vi "Práctica01_Ejercicio1_1.vi"() -> ()   [LabVIEW 2020]
panel:
  out "Boolean 5":bool
  in  "Latch Until Released\nAntes de correr el programa presionalo\ndespues correlo una sola vez y observa el resultado cambia solo si esta presionado":bool
  out "Boolean 3":bool
  in  "Latch when Released\nAntes de correr el programa presionalo\ndespues correlo una sola vez y observa el resultado cuando lo sueltas":bool
  out "Boolean":bool
  in  "Latch When Pressed \nAntes de correr el programa presionalo\ndespues correlo una sola vez y observa el resultado enclavado":bool
  out "Boolean 6":bool
  in  "Switch Until Released\nPush button, solo cambia si esta presionado":bool
  out "Boolean 4":bool
  in  "Switch when Released\nCambia cuando lo sueltas":bool
  out "Boolean 2":bool
  in  "Switch when Pressed - \nCambia cuando lo presionas":bool
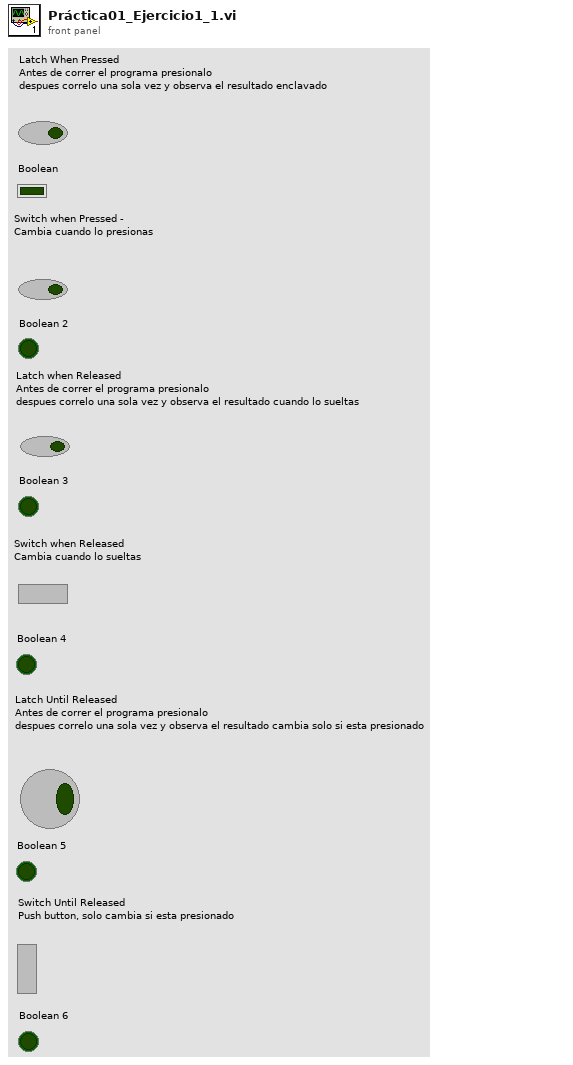
[diagram p1: front panel]
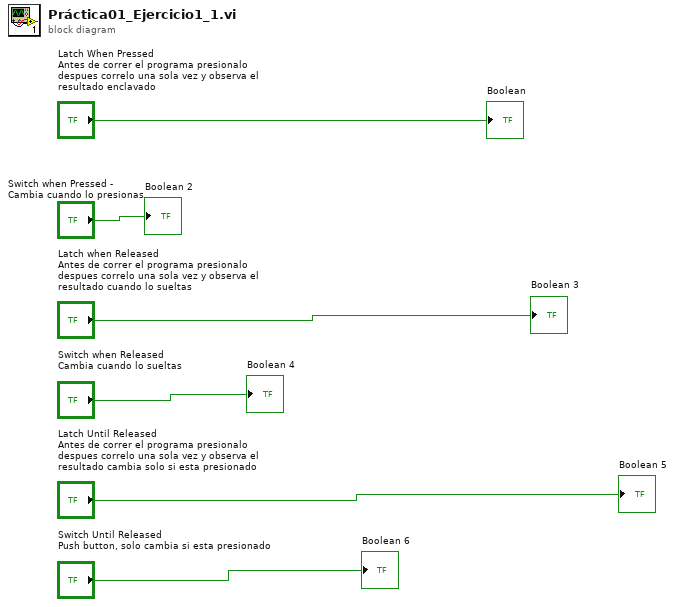
[diagram p0: block diagram]
diagram:
  "Boolean 2" <- "Switch when Pressed - \nCambia cuando lo presionas"
  "Boolean 4" <- "Switch when Released\nCambia cuando lo sueltas"
  "Boolean 6" <- "Switch Until Released\nPush button, solo cambia si esta presionado"
  "Boolean" <- "Latch When Pressed \nAntes de correr el programa presionalo\ndespues correlo una sola vez y observa el resultado enclavado"
  "Boolean 3" <- "Latch when Released\nAntes de correr el programa presionalo\ndespues correlo una sola vez y observa el resultado cuando lo sueltas"
  "Boolean 5" <- "Latch Until Released\nAntes de correr el programa presionalo\ndespues correlo una sola vez y observa el resultado cambia solo si esta presionado"
